vi "Get marker name.vi"(6 "Source VI":refnum<vi>, 7 "SPECTRUM":refnum<vi>, 8 "Text":string, 9 "Cursor Pos":cluster{"Left":i16, "Top":i16}, 10 "BW":string, 11 "Fc":string) -> (1 "cancelled":bool, 3 "text":string)   [LabVIEW 2019]
panel:
  in  "Send to Channelizer":bool
  in  "View Narrow Band":bool
  in  "Send to DF":bool
  in  "Cancel":bool
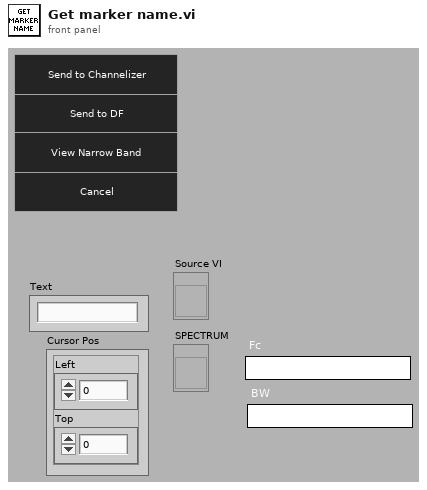
[diagram p1: front panel]
types:
  T1 = cluster{"Numeric Control":u32, "Numeric Control":u32}[]
  T2 = enum32{"Invalid", "Default", "Floating", "Floating/Auto-Hide", "Modal"}
  T3 = enum32{"Invalid", "Standard", "Closed", "Hidden", "Minimized", "Maximized"}
  T4 = typedef "LVRectTypeDef.ctl" = cluster{"Left":i16, "Top":i16, "Right":i16, "Bottom":i16}
  T5 = enum8{"Enabled", "Disabled", "Disabled and Grayed Out"}
  T6 = typedef "lveventtype.ctl" = enum32{"Null", "Timeout", "Annotation Menu Selection", "Annotation Menu Selection?", "App Instance Close", "App Instance Close?", "Autoscale Range Change", "Bookmark Info Change", "Cell Edit", "Cell Edit?", "Cursor Grab", "Cursor Grab?", "Cursor Menu Selection", "Cursor Menu Selection?", "Cursor Move", "Cursor Release", "Data Change", "Direction Change", "Display State Change", "Drag Ended", "Drag Enter", "Drag Leave", "Drag Over", "Drag Source Update", "Drag Starting", "Drag Starting?", "Drop", "Exec State Change", "Key Down", "Key Down?", "Key Repeat", "Key Repeat?", "Key Up", "Listbox Double Click", "Menu Activation?", "Menu Selection (App)", "Menu Selection? (App)", "Menu Selection (User)", "Mouse Down", "Mouse Down?", "Mouse Enter", "Mouse Leave", "Mouse Move", "Mouse Up", "Mouse Wheel", "NI Security User Change (App)", "Pane Size", "Panel Close", "Panel Close?", "Panel Resize", "Plot Attribute Change", "Scale Range Change", "Shortcut Menu Activation?", "Shortcut Menu Selection (App)", "Shortcut Menu Selection? (App)", "Shortcut Menu Selection (User)", "Tree Double Click", "Tree Drag", "Tree Drag?", "Tree Drop", "Tree Drop?", "Tree Item Close", "Tree Item Close?", "Tree Item Open", "Tree Item Open?", "User Event", "Value Change"}
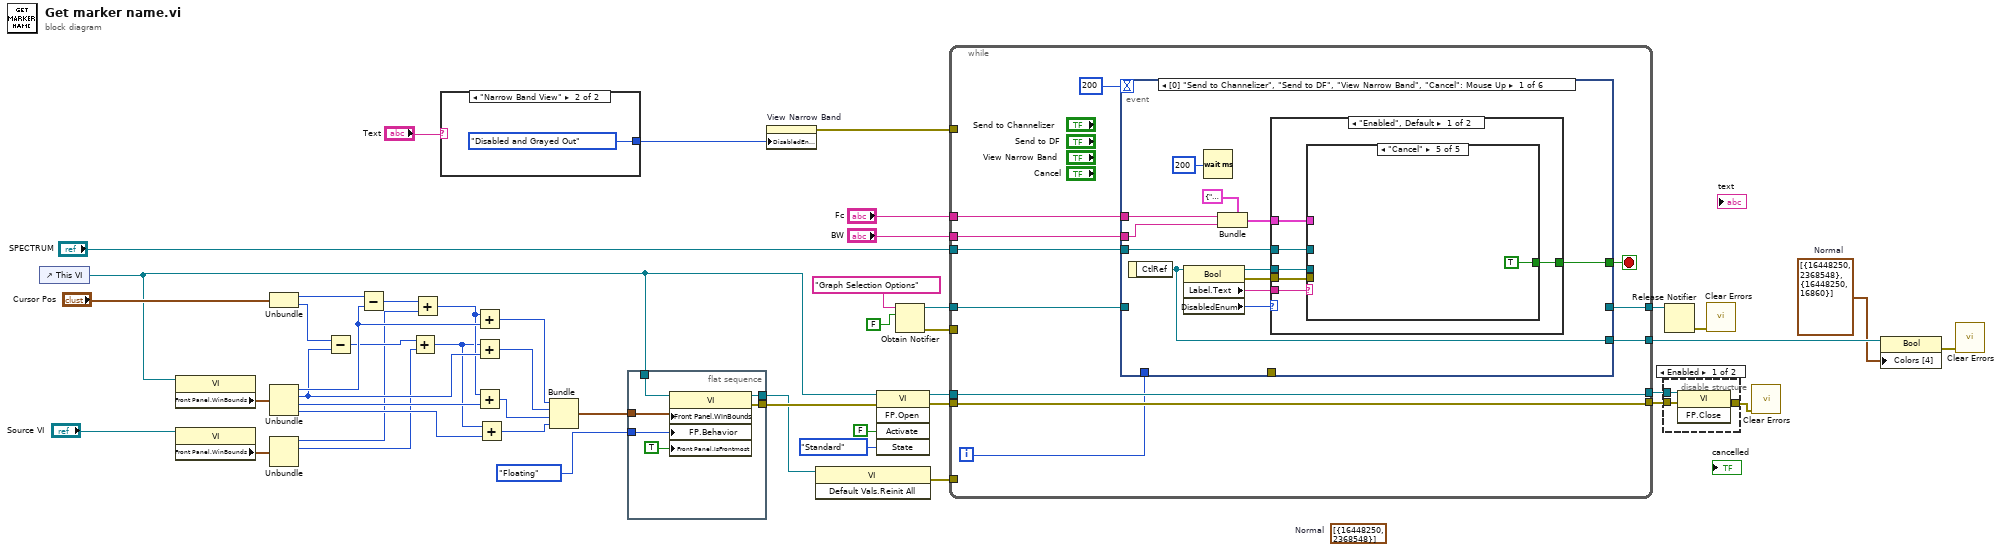
[diagram p0: block diagram]
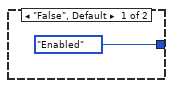
[diagram p3: hidden frame]
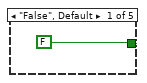
[diagram p4: hidden frame]
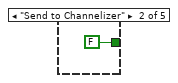
[diagram p5: hidden frame]
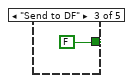
[diagram p6: hidden frame]
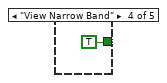
[diagram p7: hidden frame]
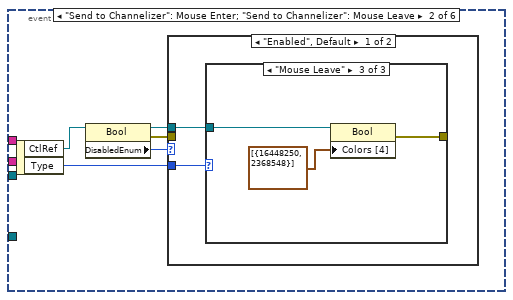
[diagram p9: hidden frame]
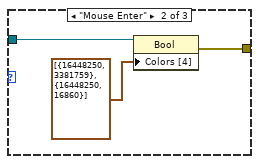
[diagram p11: hidden frame]
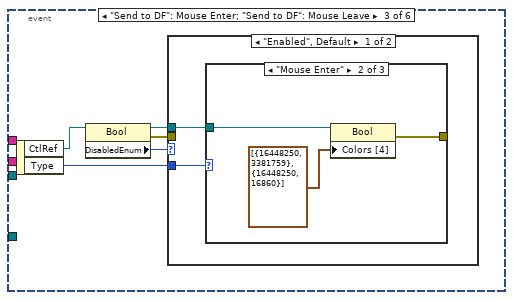
[diagram p13: hidden frame]
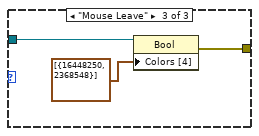
[diagram p15: hidden frame]
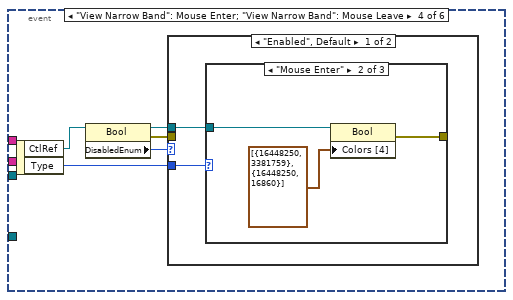
[diagram p17: hidden frame]
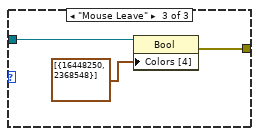
[diagram p19: hidden frame]
diagram:
  (unwired) T1 [{"Numeric Control"=16448250, "Numeric Control"=2368548}]  # Normal
  w12 = T1 [{"Numeric Control"=16448250, "Numeric Control"=2368548}, {"Numeric Control"=16448250, "Numeric Control"=16860}]  # Normal
  n1 = control-ref of="This VI"() -> (w21:refnum<vi>)
  n2 = property class="VI"(reference=w21) -> ("Front Panel.WinBounds"=w48:T4)  [unwired: 1 in, 2 out]
  n3 = property class="VI"(reference="Source VI") -> ("Front Panel.WinBounds"=w18:T4)  [unwired: 1 in, 2 out]
  n4 = Unbundle("Cursor Pos") -> ("Left"=w46:i16, "Top"=w45:i16)
  n5 = Unbundle(w48) -> ("Left"=w43:i16, "Top"=w42:i16, "Right"=w39:i16, "Bottom"=w38:i16)
  n6 = Unbundle(w18) -> ("Left"=w17:i16, "Top"=w15:i16)  [unwired: 2 out]
  n7 = Subtract(x=w45, y=w42) -> (x-y=w40:i16)
  n8 = Subtract(x=w46, y=w43) -> (x-y=w41:i16)
  n9 = Add(x=w40, y=w15) -> (x+y=w16:i16)
  n10 = Add(x=w41, y=w17) -> (x+y=w19:i16)
  n11 = case shown="\"Narrow Band View\"" "Text" {
    tunnel: [T5."Enabled" ("Disabled") T5."Disabled and Grayed Out" ("Disabled")] -> w23
    frame "False", Default {
    }
    frame "Narrow Band View" {
    }
  }
  n12 = Add(x=w19, y=w43) -> (x+y=w37:i16)
  n13 = Add(x=w16, y=w42) -> (x+y=w36:i16)
  n14 = Add(x=w19, y=w39) -> (x+y=w35:i16)
  n15 = Add(x=w16, y=w38) -> (x+y=w34:i16)
  n16 = Bundle(w37, w36, w35, w34) -> (w44:cluster{i16, i16, i16, i16})  [unwired: 1 in]
  n17 = flat-sequence {
    tunnel: w44 -> [w56]
    tunnel: [w55] -> w33
    tunnel: w21 -> [w54]
    tunnel: T2."Floating" ("Front Panel Window:Behavior") -> [w53]
    tunnel: [w52] -> w10
    frame #0 {
      n18 = property class="VI"(reference=w54, "Front Panel.WinBounds"=w56, "FP.Behavior"=w53, "Front Panel.IsFrontmost"=TRUE ("Front Panel Window:Is Frontmost")) -> (reference out=w52:refnum<vi>, error out=w55:errorcluster)  [unwired: 1 in]
    }
  }
  n19 = property on="View Narrow Band" class="Bool"("DisabledEnum"=w23) -> (error out=w22:errorcluster)  [unwired: 2 in, 1 out]
  n20 = invoke class="VI" method="Default Vals.Reinit All"(reference=w10) -> (error out=w9:errorcluster)  [unwired: 2 in, 2 out]
  n21 = invoke class="VI" method="FP.Open"(reference=w21, error in=w33, "Activate"=FALSE ("Activate?"), "State"=T3."Standard") -> (reference out=w29:refnum<vi>, error out=w30:errorcluster)  [unwired: 1 in, 3 out]
  n22 = Obtain Notifier(name (unnamed)="Graph Selection Options", notification data type=FALSE) -> (notifier out=w8:refnum<notifier>, error out=w4:errorcluster)  [unwired: 2 in, 1 out]
  n23 = while {
    tunnel: w30 -> [w66]
    tunnel: [w66] -> w27
    tunnel: w29 -> [w65]
    tunnel: [w65] -> w28
    tunnel: "SPECTRUM" -> [w64]
    tunnel: w22 -> [_]
    tunnel: [w61] -> w13
    tunnel: w9 -> [_]
    tunnel: w8 -> [w60]
    tunnel: [w59] -> w5
    tunnel: w4 -> [_]
    tunnel: "BW" -> [w58]
    tunnel: "Fc" -> [w57]
    i -> [w62]
    stop <- w67 stop-if-true
    n24 = event shown="[0] \"Send to Channelizer\", \"Send to DF\", \"View Narrow Band\", \"Cancel\": Mouse Up" {
      selector: _ -> [_ _ _ _ _ _]
      dyn-events: _ -> [_ _ _ _ _ _]
      timeout: 200 -> [_ _ _ _ _ _]
      tunnel: w58 -> [w76 _ _ _ _ _]
      tunnel: w57 -> [w77 _ _ _ _ _]
      tunnel: [w74 _ _ _ _ w145] -> w67
      tunnel: w64 -> [w71 _ _ _ _ _]
      tunnel: w62 -> [_ _ _ _ _ _]
      tunnel: [w68 _ _ _ _ _] -> w61
      tunnel: w60 -> [_ _ _ _ _ w147]
      tunnel: [_ _ _ _ _ w144] -> w59
      tunnel: [_ _ _ _ _ w143] -> _
      event "Send to Channelizer", "Send to DF", "View Narrow Band", "Cancel": Mouse Up {
        n25 = event-data() -> ("CtlRef"=w68:refnum<vi>)  [unwired: 1 in]
        n26 = property class="Bool"(reference=w68) -> (reference out=w69:refnum<vi>, error out=w73:errorcluster, "Label.Text"=w79:string, "DisabledEnum"=w70:T5)  [unwired: 1 in]
        n27 = Wait (ms)(milliseconds to wait=u32 200) -> ()  [unwired: 1 out]
        n28 = Bundle(cluster=cluster{"Fc":string, "BW":string} {"Fc"="", "BW"=""}, "Fc"=w77, "BW"=w76) -> (w75:cluster{"Fc":string, "BW":string})
        n29 = case shown="\"Enabled\", Default" w70 {
          tunnel: w79 -> [w85 _]
          tunnel: w75 -> [w84 _]
          tunnel: [w83 _] -> w74
          tunnel: w73 -> [w82 _]
          tunnel: w71 -> [w81 _]
          tunnel: w69 -> [w80 _]
          frame "Enabled", Default {
            n30 = case shown="\"Cancel\"" w85 {
              tunnel: w84 -> [_ _ _ _ _]
              tunnel: [FALSE FALSE FALSE TRUE TRUE] -> w83
              tunnel: w82 -> [_ _ _ _ _]
              tunnel: w81 -> [_ _ _ _ _]
              tunnel: w80 -> [_ _ _ _ _]
              frame "False", Default {
              }
              frame "Send to Channelizer" {
              }
              frame "Send to DF" {
              }
              frame "View Narrow Band" {
              }
              frame "Cancel" {
              }
            }
          }
          frame "Disabled", "Disabled and Grayed Out" {
          }
        }
      }
      event "Send to Channelizer": Mouse Enter; "Send to Channelizer": Mouse Leave {
        n31 = event-data() -> ("CtlRef"=w93:refnum<vi>, "Type"=w94:T6)  [unwired: 1 in]
        n32 = property class="Bool"(reference=w93) -> (reference out=w92:refnum<vi>, error out=w91:errorcluster, "DisabledEnum"=w95:T5)  [unwired: 1 in]
        n33 = case shown="\"Enabled\", Default" w95 {
          tunnel: w94 -> [w97 _]
          tunnel: w92 -> [w96 _]
          tunnel: w91 -> [_ _]
          frame "Enabled", Default {
            n34 = case shown="\"Mouse Leave\"" w97 {
              tunnel: w96 -> [_ w100 w103]
              tunnel: [_ w98 w102] -> _
              frame Default {
              }
              frame "Mouse Enter" {
                n35 = property class="Bool"(reference=w100, "Colors [4]"=T1 [{"Numeric Control"=16448250, "Numeric Control"=3381759}, {"Numeric Control"=16448250, "Numeric Control"=16860}]) -> (error out=w98:errorcluster)  [unwired: 1 in, 1 out]
              }
              frame "Mouse Leave" {
                n36 = property class="Bool"(reference=w103, "Colors [4]"=T1 [{"Numeric Control"=16448250, "Numeric Control"=2368548}]) -> (error out=w102:errorcluster)  [unwired: 1 in, 1 out]
              }
            }
          }
          frame "Disabled", "Disabled and Grayed Out" {
          }
        }
      }
      event "Send to DF": Mouse Enter; "Send to DF": Mouse Leave {
        n37 = event-data() -> ("CtlRef"=w106:refnum<vi>, "Type"=w107:T6)  [unwired: 1 in]
        n38 = property class="Bool"(reference=w106) -> (reference out=w105:refnum<vi>, error out=w104:errorcluster, "DisabledEnum"=w108:T5)  [unwired: 1 in]
        n39 = case shown="\"Enabled\", Default" w108 {
          tunnel: w107 -> [w110 _]
          tunnel: w105 -> [w109 _]
          tunnel: w104 -> [_ _]
          frame "Enabled", Default {
            n40 = case shown="\"Mouse Enter\"" w110 {
              tunnel: w109 -> [_ w113 w116]
              tunnel: [_ w111 w115] -> _
              frame Default {
              }
              frame "Mouse Enter" {
                n41 = property class="Bool"(reference=w113, "Colors [4]"=T1 [{"Numeric Control"=16448250, "Numeric Control"=3381759}, {"Numeric Control"=16448250, "Numeric Control"=16860}]) -> (error out=w111:errorcluster)  [unwired: 1 in, 1 out]
              }
              frame "Mouse Leave" {
                n42 = property class="Bool"(reference=w116, "Colors [4]"=T1 [{"Numeric Control"=16448250, "Numeric Control"=2368548}]) -> (error out=w115:errorcluster)  [unwired: 1 in, 1 out]
              }
            }
          }
          frame "Disabled", "Disabled and Grayed Out" {
          }
        }
      }
      event "View Narrow Band": Mouse Enter; "View Narrow Band": Mouse Leave {
        n43 = event-data() -> ("CtlRef"=w119:refnum<vi>, "Type"=w120:T6)  [unwired: 1 in]
        n44 = property class="Bool"(reference=w119) -> (reference out=w118:refnum<vi>, error out=w117:errorcluster, "DisabledEnum"=w121:T5)  [unwired: 1 in]
        n45 = case shown="\"Enabled\", Default" w121 {
          tunnel: w120 -> [w123 _]
          tunnel: w118 -> [w122 _]
          tunnel: w117 -> [_ _]
          frame "Enabled", Default {
            n46 = case shown="\"Mouse Enter\"" w123 {
              tunnel: w122 -> [_ w126 w129]
              tunnel: [_ w124 w128] -> _
              frame Default {
              }
              frame "Mouse Enter" {
                n47 = property class="Bool"(reference=w126, "Colors [4]"=T1 [{"Numeric Control"=16448250, "Numeric Control"=3381759}, {"Numeric Control"=16448250, "Numeric Control"=16860}]) -> (error out=w124:errorcluster)  [unwired: 1 in, 1 out]
              }
              frame "Mouse Leave" {
                n48 = property class="Bool"(reference=w129, "Colors [4]"=T1 [{"Numeric Control"=16448250, "Numeric Control"=2368548}]) -> (error out=w128:errorcluster)  [unwired: 1 in, 1 out]
              }
            }
          }
          frame "Disabled", "Disabled and Grayed Out" {
          }
        }
      }
      event "Cancel": Mouse Enter; "Cancel": Mouse Leave {
        n49 = event-data() -> ("CtlRef"=w132:refnum<vi>, "Type"=w133:T6)  [unwired: 1 in]
        n50 = property class="Bool"(reference=w132) -> (reference out=w131:refnum<vi>, error out=w130:errorcluster, "DisabledEnum"=w134:T5)  [unwired: 1 in]
        n51 = case shown="\"Enabled\", Default" w134 {
          tunnel: w133 -> [w136 _]
          tunnel: w131 -> [w135 _]
          tunnel: w130 -> [_ _]
          frame "Enabled", Default {
            n52 = case shown="\"Mouse Leave\"" w136 {
              tunnel: w135 -> [_ w139 w142]
              tunnel: [_ w137 w141] -> _
              frame Default {
              }
              frame "Mouse Enter" {
                n53 = property class="Bool"(reference=w139, "Colors [4]"=T1 [{"Numeric Control"=16448250, "Numeric Control"=3381759}, {"Numeric Control"=16448250, "Numeric Control"=16860}]) -> (error out=w137:errorcluster)  [unwired: 1 in, 1 out]
              }
              frame "Mouse Leave" {
                n54 = property class="Bool"(reference=w142, "Colors [4]"=T1 [{"Numeric Control"=16448250, "Numeric Control"=2368548}]) -> (error out=w141:errorcluster)  [unwired: 1 in, 1 out]
              }
            }
          }
          frame "Disabled", "Disabled and Grayed Out" {
          }
        }
      }
      event Timeout {
        n55 = event-data() -> ()  [unwired: 1 in, 3 out]
        n56 = Wait on Notification(notifier=w147, timeout in ms (-1)=10) -> (notifier out=w144:refnum<notifier>, notification=w145:bool, error out=w143:errorcluster)  [unwired: 2 in, 1 out]
      }
    }
  }
  n57 = disable-structure shown="Enabled" {
    disable-tunnel: w28 -> [w150 _]
    disable-tunnel: w27 -> [w149 w151]
    disable-tunnel: [w148 w151] -> w26
    frame Enabled {
      n58 = invoke class="VI" method="FP.Close"(reference=w150, error in=w149) -> (error out=w148:errorcluster)  [unwired: 1 in, 2 out]
    }
    frame Disabled {
    }
  }
  n59 = Release Notifier(notifier=w5) -> (error out=w3:errorcluster)  [unwired: 2 in, 2 out]
  n60 = call <vilib>:"Clear Errors.vi"("error in (no error)"=w3) -> ()  [unwired: 5 in, 2 out]
  n61 = call <vilib>:"Clear Errors.vi"("error in (no error)"=w26) -> ()  [unwired: 5 in, 2 out]
  n62 = property class="Bool"(reference=w13, "Colors [4]"=w12) -> (error out=w11:errorcluster)  [unwired: 1 in, 1 out]
  n63 = call <vilib>:"Clear Errors.vi"("error in (no error)"=w11) -> ()  [unwired: 5 in, 2 out]
